vi "Get Segment.vi"(8 "error in (no error)":errorcluster, 10 "Segment index":i32, 11 "TreeNode in":refnum<class "TreeNode.lvclass">) -> (0 "error out":errorcluster, 2 "Data out":refnum<class "Array.lvclass">, 3 "TreeNode out":refnum<class "TreeNode.lvclass">)   [LabVIEW 2015, in "MDSplus.lvlib" / "TreeNode.lvclass"]
doc: "Get data form the selected segment."
uses:
  <vilib>/MDSplus/Classes/Data_Class/TreeNode_Class/TreeNode.lvclass
  <vilib>/MDSplus/Classes/Data_Class/Array_Class/Array.lvclass
  <vilib>/MDSplus/Classes/Data_Class/Data.lvclass
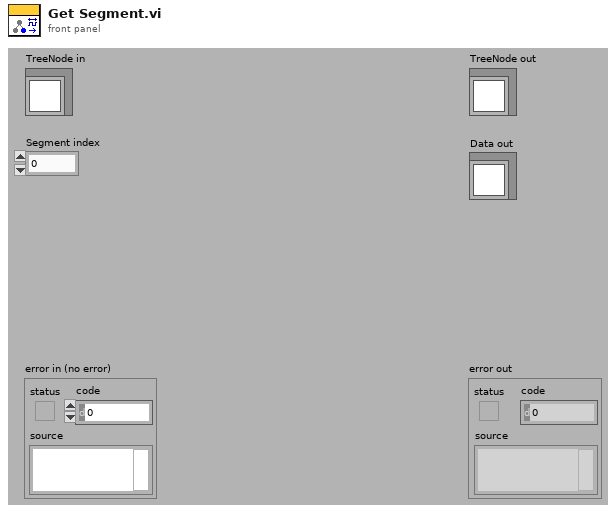
[diagram p1: front panel]
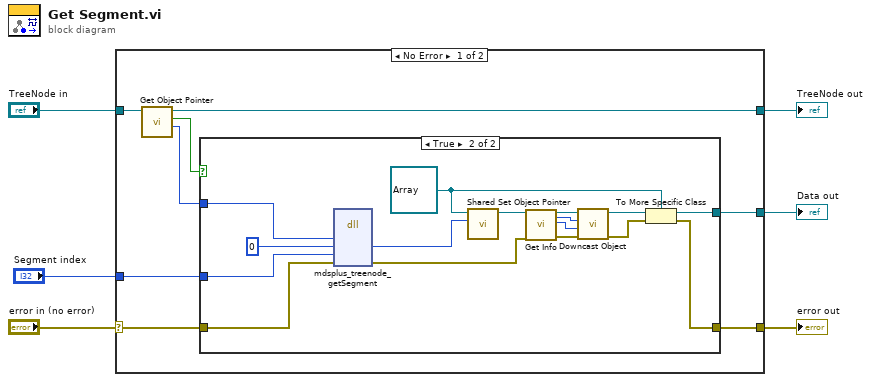
[diagram p0: block diagram]
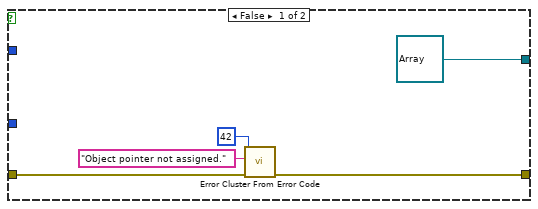
[diagram p2: hidden frame]
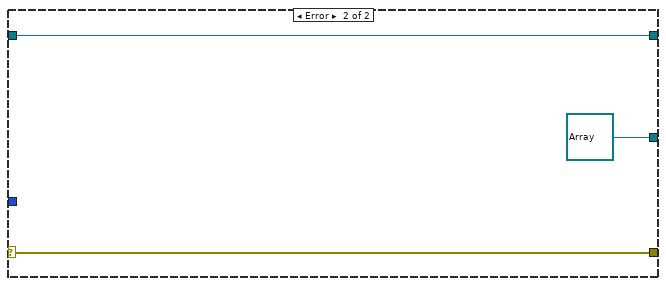
[diagram p3: hidden frame]
diagram:
  n1 = case shown="No Error" "error in (no error)" {
    selector: "error in (no error)" -> [w10 w38]
    tunnel: [w9 w38] -> w5
    tunnel: [w8 w37] -> w3
    tunnel: "TreeNode in" -> [w13 w37]
    tunnel: [w14 refnum<class "Array.lvclass"> refnum ("Data out")] -> w2
    tunnel: "Segment index" -> [w7 _]
    frame No Error {
      n2 = call-dynamic "Get Object Pointer.vi"("Data in"=w13) -> ("Object Pointer"=w11:i64, "Assigned object pointer?"=w12:bool, "Data out"=w8:refnum<class "TreeNode.lvclass">)  [unwired: 8 in]
      n3 = case shown="True" w12 {
        tunnel: [refnum<class "Array.lvclass"> refnum ("Data out") w24] -> w14
        tunnel: w11 -> [_ w28]
        tunnel: w10 -> [w16 w26]
        tunnel: [w15 w22] -> w9
        tunnel: w7 -> [_ w20]
        frame False {
          n4 = call <vilib>:"Error Cluster From Error Code.vi"("error in (no error)"=w16, "error message (\"\")"="Object pointer not assigned." ("error message (\"\")"), "error code (0)"=42) -> ("error out"=w15:errorcluster)  [unwired: 6 in]
        }
        frame True {
          w21 = refnum<class "Array.lvclass"> refnum ("Array.lvclass")
          n5 = dll-call lib="MDSobjectsLVShr" fn="mdsplus_treenode_getSegment"("lvTreeNodePtr"=w28, "lvArrayPtrOut"=i64 0 ("lvDataPtrOut"), "segIdxIn"=w20, "error"=w26) -> ("lvArrayPtrOut"=w34:i64, "error"=w27:errorcluster)  [unwired: 6 in, 2 out]
          n6 = call <vilib>:"Shared Set Object Pointer.vi"("Object Pointer"=w34, "Data in"=w21) -> ("Data out"=w33:refnum<class "Array.lvclass">)  [unwired: 9 in]
          n7 = call-dynamic "Get Info.vi"("Array in"=w33, "error in (no error)"=w27) -> ("Array out"=w32:refnum<class "Array.lvclass">, "Class type out"=w31:u8, "Data type out"=w30:u8, "error out"=w29:errorcluster)  [unwired: 12 in, 2 out]
          n8 = call <vilib>:"Downcast Object.vi"("error in (no error)"=w29, "Data Type"=w30, "Class Type"=w31, "Data in"=w32) -> ("error out"=w23:errorcluster, "Data out"=w25:refnum<class "Data.lvclass">)  [unwired: 6 in]
          n9 = To More Specific Class(target class=w21, reference=w25, error in=w23) -> (specific class reference=w24:refnum<class "Array.lvclass">, error out=w22:errorcluster)
        }
      }
    }
    frame Error {
    }
  }
  "error out" <- w5
  "TreeNode out" <- w3
  "Data out" <- w2
